vi "enumerate_structuring_elements.vi"(4 "Rotational and Refelective Invariance (T)":bool=TRUE, 5 "Structuring Elements":i32[][][](array[numeric])=[[[1, 1, 1], [1, 1, 1], [1, 1, 1]]]) -> (2 "Enumerated Structuring Elements":i32[][][](array[numeric]))   [LabVIEW 2019]
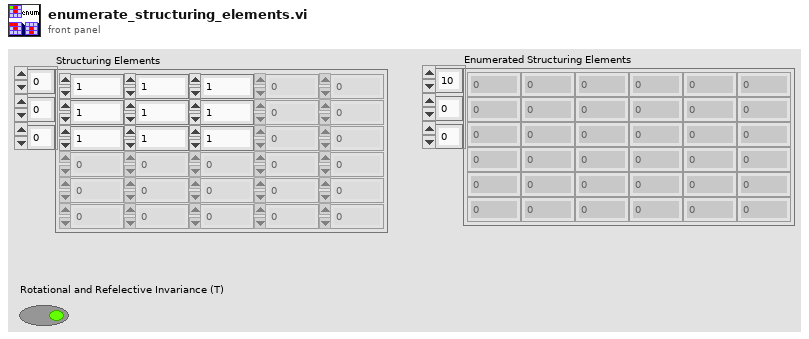
[diagram p1: front panel]
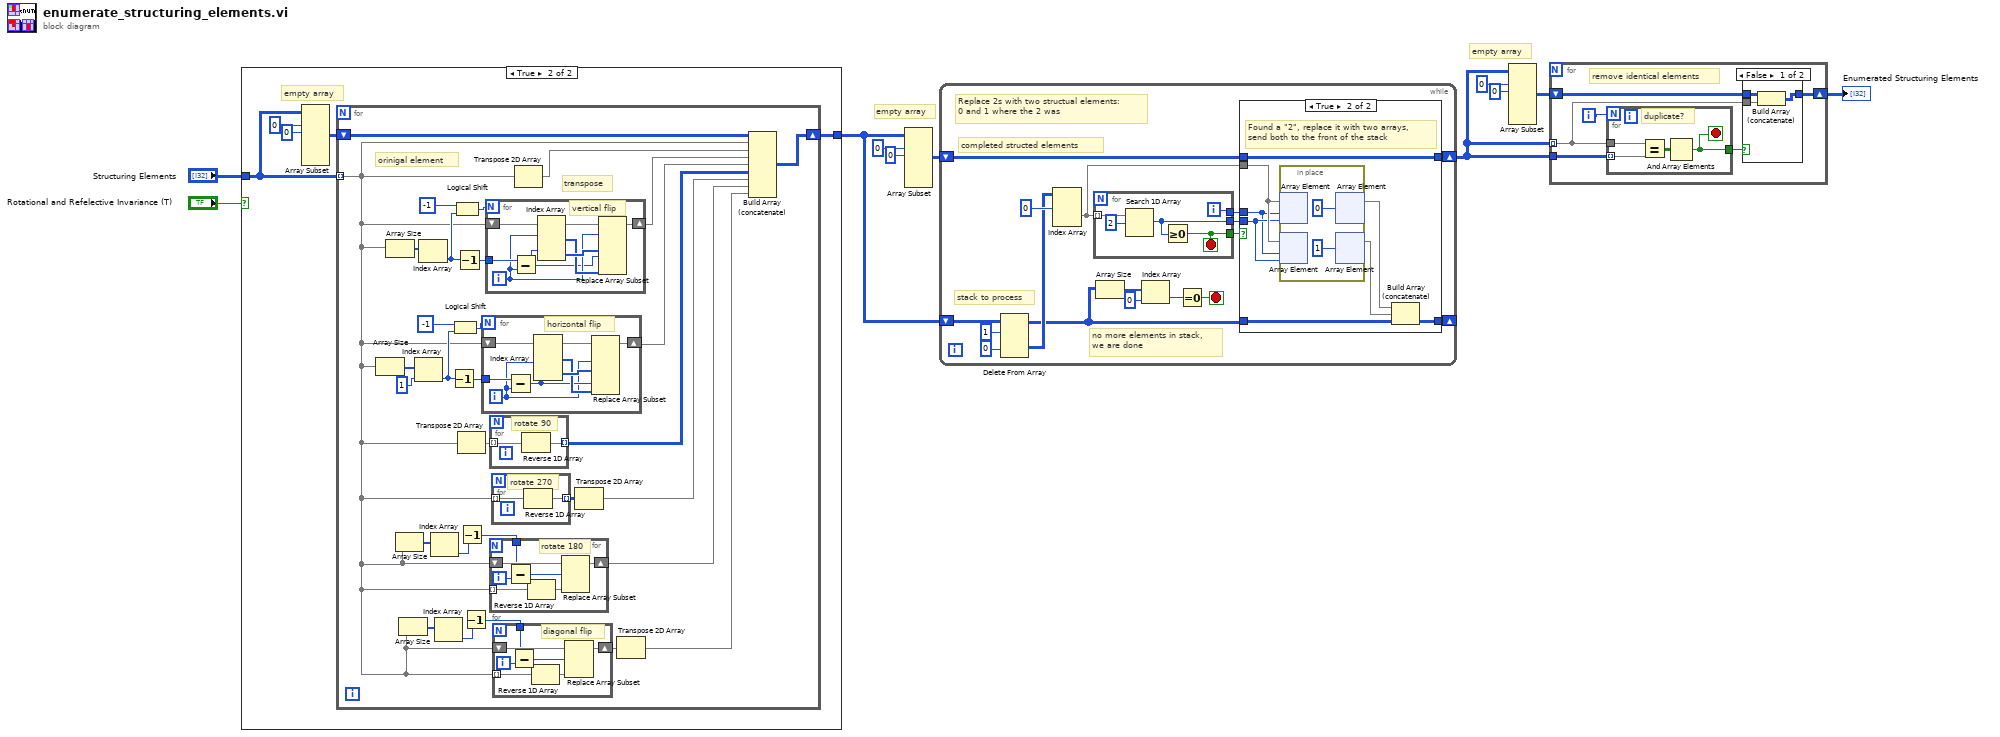
[diagram p0: block diagram]
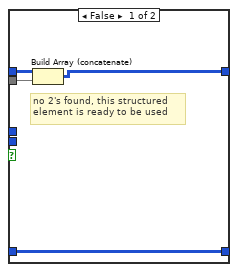
[diagram p2: hidden frame]
diagram:
  # "empty array"
  # "empty array"
  n1 = case shown="True" "Rotational and Refelective Invariance (T)" {
    tunnel: "Structuring Elements" -> [w12 w15]
    tunnel: [w12 w13] -> w3
    frame False {
    }
    frame True {
      # "empty array"
      n2 = Array Subset(array=w15, index (dim 0)=0 ("index"), length (dim 0)=0 ("length")) -> (w14:i32[][][])  [unwired: 4 in]
      n3 = for {
        tunnel: w15 -> [w26] mode=indexing
        shift-right: [w18] -> w13
        shift-left: w14 -> [w27]
        # "orinigal element"
        # "transpose"
        n4 = Array Size(array=w26) -> (size(s)=w37:i32[])
        n5 = Array Size(array=w26) -> (size(s)=w46:i32[])
        n6 = Array Size(array=w26) -> (size(s)=w34:i32[])
        n7 = Array Size(array=w26) -> (size(s)=w29:i32[])
        n8 = Index Array(array=w37, index=1) -> (element=w39:i32)
        n9 = Index Array(array=w46) -> (element=w44:i32)  [unwired: 1 in]
        n10 = Index Array(array=w34) -> (element=w32:i32)  [unwired: 1 in]
        n11 = Index Array(array=w29) -> (element=w31:i32)  [unwired: 1 in]
        n12 = Decrement(x=w39) -> (x-1=w41:i32)
        n13 = Logical Shift(y=i8 -1, x=w39) -> (x << y=w38:i32)
        n14 = Logical Shift(y=i8 -1, x=w44) -> (x << y=w45:i32)
        n15 = Decrement(x=w44) -> (x-1=w42:i32)
        n16 = Transpose 2D Array(2D array=w26) -> (transposed array=w36:i32[][])
        n17 = Decrement(x=w32) -> (x-1=w33:i32)
        n18 = Decrement(x=w31) -> (x-1=w30:i32)
        n19 = for {
          N: w38 -> [_]
          shift-right: [w68] -> w23
          shift-left: w26 -> [w67]
          tunnel: w41 -> [w64]
          i -> [w62]
          # "horizontal flip"
          n20 = Subtract(x=w64, y=w62) -> (x-y=w63:i32)
          n21 = Index Array(array=w67, index (col) #1=w62, index (col) #2=w63) -> (element #1=w65:i32[], element #2=w66:i32[])  [unwired: 2 in]
          n22 = Replace Array Subset(array=w67, new element #1=w66, index (col) #1=w62, new element #2=w65, index (col) #2=w63) -> (w68:i32[][])  [unwired: 2 in]
        }
        n23 = for {
          N: w45 -> [_]
          shift-right: [w79] -> w24
          shift-left: w26 -> [w78]
          tunnel: w42 -> [w75]
          i -> [w74]
          # "vertical flip"
          n24 = Subtract(x=w75, y=w74) -> (x-y=w73:i32)
          n25 = Index Array(array=w78, index (row) #1=w74, index (row) #2=w73) -> (element #1=w76:i32[], element #2=w77:i32[])  [unwired: 2 in]
          n26 = Replace Array Subset(array=w78, new element #1=w77, index (row) #1=w74, new element #2=w76, index (row) #2=w73) -> (w79:i32[][])  [unwired: 2 in]
        }
        n27 = for {
          shift-right: [w61] -> w20
          shift-left: w26 -> [w60]
          tunnel: w33 -> [w58]
          tunnel: w26 -> [w55] mode=indexing
          i -> [w59]
          # "rotate 180"
          n28 = Subtract(x=w58, y=w59) -> (x-y=w57:i32)
          n29 = Reverse 1D Array(array=w55) -> (reversed array=w56:i32[])
          n30 = Replace Array Subset(array=w60, new element=w56, index (row)=w57) -> (w61:i32[][])  [unwired: 1 in]
        }
        n31 = for {
          tunnel: w36 -> [w72] mode=indexing
          tunnel: [w71] -> w22 mode=indexing
          # "rotate 90"
          n32 = Reverse 1D Array(array=w72) -> (reversed array=w71:i32[])
        }
        n33 = for {
          tunnel: w26 -> [w70] mode=indexing
          tunnel: [w69] -> w47 mode=indexing
          # "rotate 270"
          n34 = Reverse 1D Array(array=w70) -> (reversed array=w69:i32[])
        }
        n35 = for {
          shift-right: [w54] -> w28
          shift-left: w26 -> [w53]
          tunnel: w30 -> [w51]
          tunnel: w26 -> [w48] mode=indexing
          i -> [w52]
          # "diagonal flip"
          n36 = Subtract(x=w51, y=w52) -> (x-y=w50:i32)
          n37 = Reverse 1D Array(array=w48) -> (reversed array=w49:i32[])
          n38 = Replace Array Subset(array=w53, new element=w49, index (row)=w50) -> (w54:i32[][])  [unwired: 1 in]
        }
        n39 = Transpose 2D Array(2D array=w26) -> (transposed array=w25:i32[][])
        n40 = Transpose 2D Array(2D array=w47) -> (transposed array=w21:i32[][])
        n41 = Transpose 2D Array(2D array=w28) -> (transposed array=w19:i32[][])
        n42 = Build Array (concatenate)(w27, w26, w25, w24, w23, w22, w21, w20, w19) -> (w18:i32[][][])
      }
    }
  }
  n43 = Array Subset(array=w3, index (dim 0)=0 ("index"), length (dim 0)=0 ("length")) -> (w2:i32[][][])  [unwired: 4 in]
  n44 = while {
    shift-right: [w90] -> w1
    shift-left: w2 -> [w91]
    shift-right: [w89] -> _
    shift-left: w3 -> [w86]
    stop <- w93 stop-if-true
    # "Replace 2s with two structual elements:\n0 and 1 where the 2 was"
    # "no more elements in stack,\nwe are done"
    # "completed structed elements"
    # "stack to process"
    n45 = Delete From Array(array=w86, length=1, index (dim 0)=0 ("index (page)")) -> (deleted portion=w84:i32[][][], array with subset deleted=w80:i32[][][])  [unwired: 2 in]
    n46 = Index Array(array=w84, index (dim 0)=0 ("index")) -> (element=w81:i32[][])  [unwired: 2 in]
    n47 = for {
      tunnel: w81 -> [w115] mode=indexing
      tunnel: [w113] -> w82
      tunnel: [w112] -> w83
      tunnel: [w111] -> w92
      i -> [w112]
      stop <- w111 stop-if-true
      n48 = Search 1D Array(1D array=w115, element=2) -> (index of element=w113:i32)  [unwired: 1 in]
      n49 = Greater Or Equal To 0?(x=w113) -> (x >= 0?=w111:bool)
    }
    n50 = Array Size(array=w80) -> (size(s)=w96:i32[])
    n51 = Index Array(array=w96, index=0) -> (element=w94:i32)
    n52 = Equal To 0?(x=w94) -> (x = 0?=w93:bool)
    n53 = case shown="True" w92 {
      tunnel: w91 -> [w100 w108]
      tunnel: [w99 w108] -> w90
      tunnel: w81 -> [w98 w107]
      tunnel: [w97 w103] -> w89
      tunnel: w80 -> [w97 w104]
      tunnel: w83 -> [_ w105]
      tunnel: w82 -> [_ w106]
      frame False {
        # "no 2's found, this structured \nelement is ready to be used"
        n54 = Build Array (concatenate)(w100, w98) -> (w99:i32[][][])
      }
      frame True {
        # "Found a \"2\", replace it with two arrays, \nsend both to the front of the stack"
        n55 = in-place {
          n56 = in-place-array #1(w107, w105, w106) -> ()  [unwired: 1 out]
          n57 = in-place-array #2(w107, w105, w106) -> ()  [unwired: 1 out]
          n58 = in-place-array #1(0 ("element")) -> (w102:i32[][])  [unwired: 2 out]
          n59 = in-place-array #2(1 ("element")) -> (w101:i32[][])  [unwired: 2 out]
        }
        n60 = Build Array (concatenate)(w102, w101, w104) -> (w103:i32[][][])
      }
    }
  }
  n61 = Array Subset(array=w1, index (dim 0)=0 ("index"), length (dim 0)=0 ("length")) -> (w7:i32[][][])  [unwired: 4 in]
  n62 = for {
    tunnel: w1 -> [w117] mode=indexing
    shift-right: [w118] -> w6
    shift-left: w7 -> [w119]
    tunnel: w1 -> [w120]
    i -> [w121]
    # "remove identical elements"
    n63 = for {
      N: w121 -> [_]
      tunnel: w117 -> [w129]
      tunnel: w120 -> [w128] mode=indexing
      tunnel: [w126] -> w116
      stop <- w126 stop-if-true
      # "duplicate?"
      n64 = Equal?(x=w129, y=w128) -> (x = y?=w127:bool[][])
      n65 = And Array Elements(Boolean array=w127) -> (logical AND=w126:bool)
    }
    n66 = case shown="False" w116 {
      tunnel: w119 -> [w124 w125]
      tunnel: [w123 w125] -> w118
      tunnel: w117 -> [w122 _]
      frame False {
        n67 = Build Array (concatenate)(w124, w122) -> (w123:i32[][][])
      }
      frame True {
      }
    }
  }
  "Enumerated Structuring Elements" <- w6
